vi "Spawn.vi"(11 "TEMPLATE Actor in":refnum<class "TEMPLATE Actor.lvclass">) -> (0 "Error out":errorcluster, 3 "TEMPLATE Actor out":refnum<class "TEMPLATE Actor.lvclass">)   [LabVIEW 2020, in "_Template.lvlib" / "Templates.lvlib" / "TEMPLATE jettl Actor.lvlib" / "TEMPLATE Actor.lvlib" / "TEMPLATE Actor.lvclass"]
uses:
  TEMPLATE Actor.lvclass
  TEMPLATE Actor.lvclass/TEMPLATE Actor.ctl
  jettl/jettl/jettl.lvlib
panel:
  # "This front panel should not be manipulated."
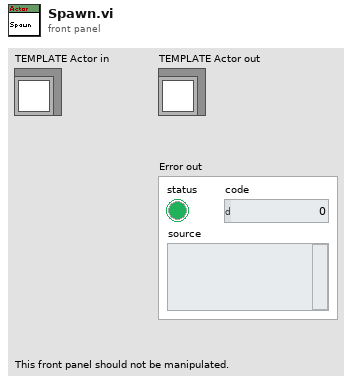
[diagram p1: front panel]
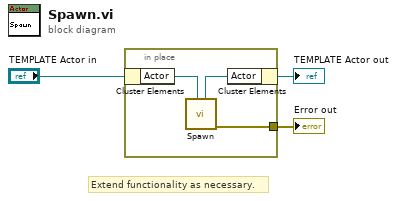
[diagram p0: block diagram]
diagram:
  # "Extend functionality as necessary."
  n1 = in-place {
    in-place-border: [w4] -> w1
    n2 = in-place-cluster #1("TEMPLATE Actor in") -> ("Actor"=w6:refnum<data-value>)
    n3 = call "Spawn.vi"("Actor in"=w6) -> ("Error out"=w4:errorcluster, "Actor out"=w5:refnum<data-value>)  [unwired: 9 in]
    n4 = in-place-cluster #1("Actor"=w5) -> (→"TEMPLATE Actor out":refnum<class "TEMPLATE Actor.lvclass">)
  }
  "Error out" <- w1
